vi "GetEnumEntrySymbolic.vi"(8 "error in (no error)":errorcluster caption="错误输入（无错误）", 9 "nValue":u32, 10 "strKey":string, 11 "handle":u64) -> (0 "error out":errorcluster caption="错误输出", 1 "EnumEntry":T1, 2 "function return":i32, 3 "handle out":u64)   [LabVIEW 2013, in "MvCameraControl.lvlib"]
doc: "MV_LV_API int __stdcall GetStringValue( void* handle, const char* strKey, MVCC_STRINGVALUE *pStringValue);"
uses:
  MvCameraControl.lvlib
  MvCameraPatch.dll
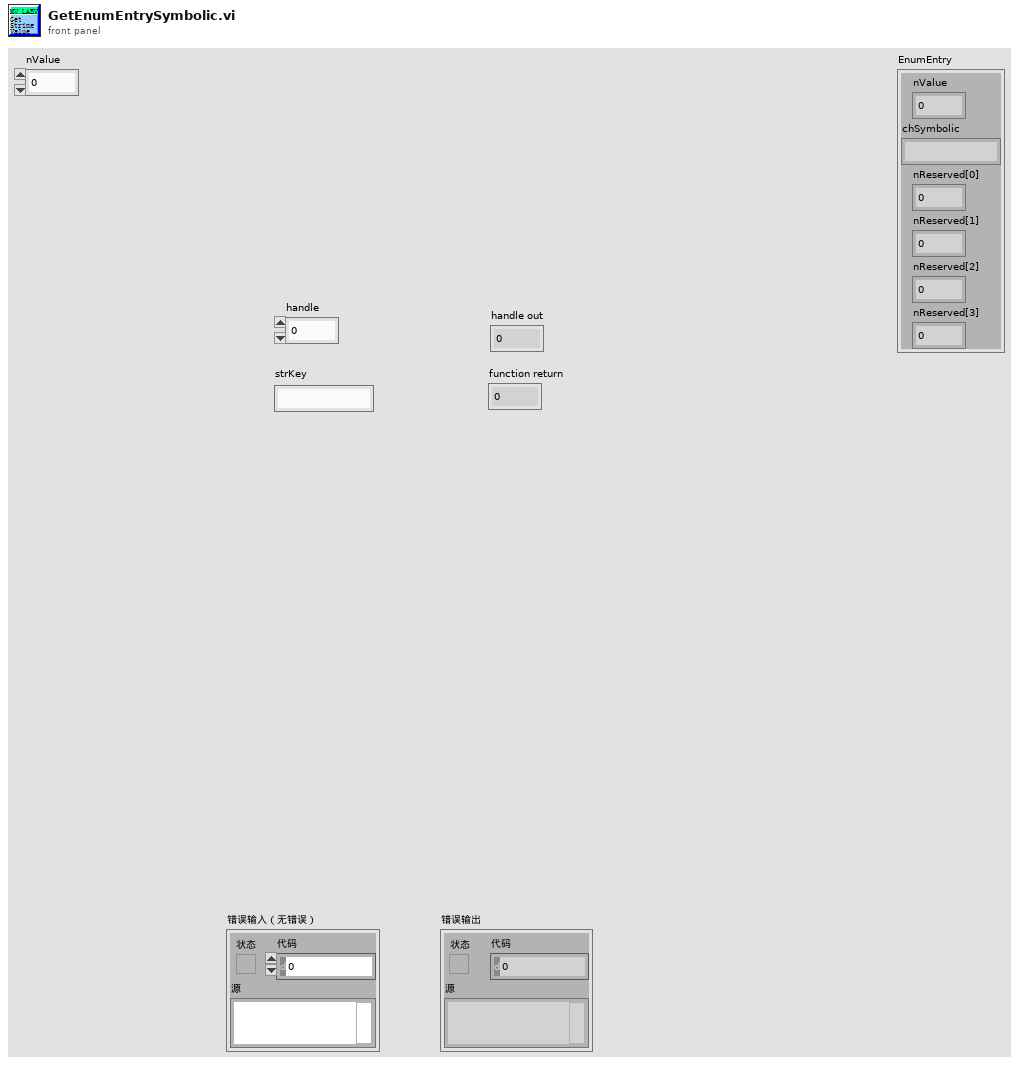
[diagram p1: front panel]
types:
  T1 = cluster{"nValue":u32, "chSymbolic":string, "nReserved[0]":u32, "nReserved[1]":u32, "nReserved[2]":u32, "nReserved[3]":u32}
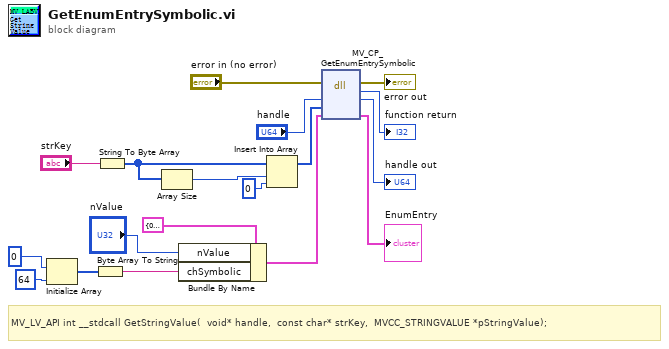
[diagram p0: block diagram]
diagram:
  # "MV_LV_API int __stdcall GetStringValue(  void* handle,  const char* strKey,  MVCC_STRINGVALUE *pStringValue);"
  n1 = Initialize Array(u8 0 ("元素"), 64 ("维数大小")) -> (w8:u8[])
  n2 = Byte Array To String(unsigned byte array=w8) -> (string=w9:string)
  n3 = String To Byte Array(string="strKey") -> (unsigned byte array=w14:u8[])
  n4 = Array Size(array=w14) -> (size(s)=w13:i32)
  n5 = Bundle By Name(cluster=T1 {"nValue"=0, "chSymbolic"="", "nReserved[0]"=0, "nReserved[1]"=0, "nReserved[2]"=0, "nReserved[3]"=0} ("EnumEntry"), "nValue"="nValue", "chSymbolic"=w9) -> (w5:T1)
  n6 = Insert Into Array(array=w14, index=w13, new element=u8 0 ("新元素/子数组")) -> (w10:u8[])
  n7 = dll-call lib="MvCameraPatch.dll" fn="MV_CP_GetEnumEntrySymbolic"(error in="error in (no error)", "handle"="handle", "strKey"=w10, "pEnumEntryValue"=w5) -> (error out=→"error out":errorcluster, "返回类型"=→"function return":i32, "handle"=→"handle out":u64, "pEnumEntryValue"=→"EnumEntry":T1)  [unwired: 3 in, 1 out]
